vi "Motion-Energize-Drives.vi"(8 "error in (no error)":errorcluster, 11 "Motion-ControlAll in":refnum<class "Motion-ControlAll.lvclass">) -> (0 "error out":errorcluster, 3 "Motion-ControlAll out":refnum<class "Motion-ControlAll.lvclass">)   [LabVIEW 2013, in "Motion-ControlAll.lvclass"]
uses:
  Motion-ControlAll.lvclass
  Motion-ControlAll.lvclass/Motion-ControlAll.ctl
  <vilib>/addons/_LabVIEW Style Book/Utilities/Style Book Utilities.lvlib
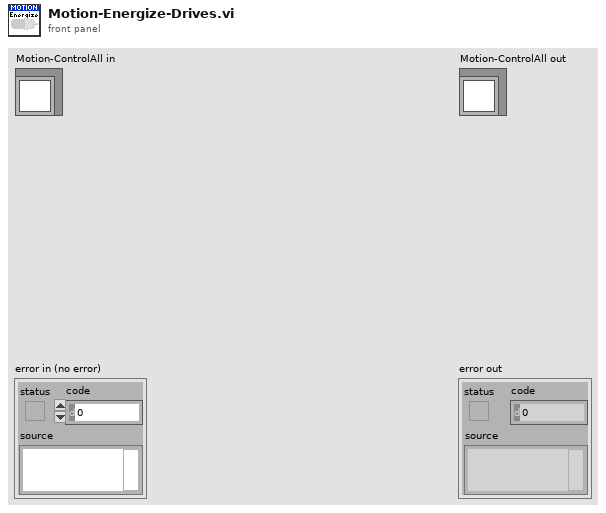
[diagram p1: front panel]
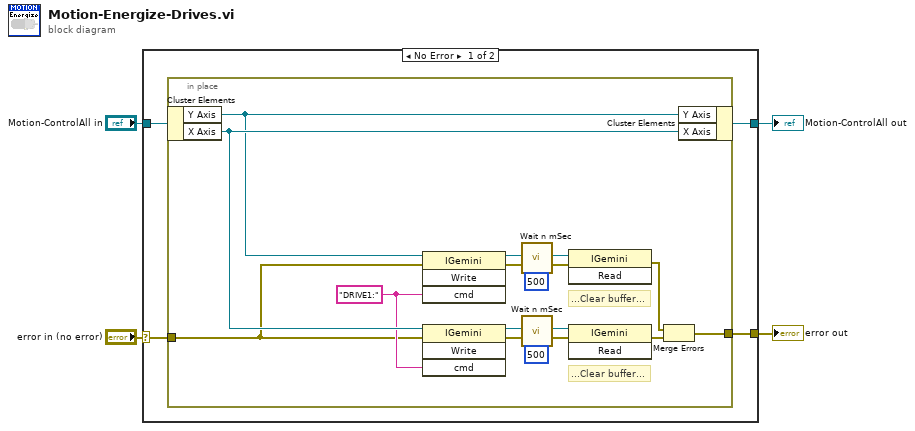
[diagram p0: block diagram]
diagram:
  n1 = case shown="No Error" "error in (no error)" {
    selector: "error in (no error)" -> [w7 w25]
    tunnel: [w6 w25] -> w3
    tunnel: [w5 w24] -> w1
    tunnel: "Motion-ControlAll in" -> [w8 w24]
    frame No Error {
      n2 = in-place {
        in-place-border: w7 -> [w20]
        in-place-border: [w9] -> w6
        w21 = "DRIVE1:"
        # "...Clear buffer..."
        # "...Clear buffer..."
        n3 = in-place-cluster #1(w8) -> ("Y Axis"=w22:refnum<k7>, "X Axis"=w23:refnum<k7>)
        n4 = invoke class="IGemini" method="Write"(reference=w22, error in=w20, "cmd"=w21) -> (reference out=w16:refnum<k7>, error out=w17:errorcluster)  [unwired: 1 in, 2 out]
        n5 = invoke class="IGemini" method="Write"(reference=w23, error in=w20, "cmd"=w21) -> (reference out=w10:refnum<k7>, error out=w12:errorcluster)  [unwired: 1 in, 2 out]
        n6 = call <vilib>:"Wait n mSec.vi"("error in (no error)"=w17, "Milliseconds to Wait (500)"=u32 500) -> ("error out"=w15:errorcluster)  [unwired: 13 in]
        n7 = call <vilib>:"Wait n mSec.vi"("error in (no error)"=w12, "Milliseconds to Wait (500)"=u32 500) -> ("error out"=w11:errorcluster)  [unwired: 13 in]
        n8 = invoke class="IGemini" method="Read"(reference=w16, error in=w15) -> (error out=w18:errorcluster)  [unwired: 1 in, 2 out]
        n9 = invoke class="IGemini" method="Read"(reference=w10, error in=w11) -> (error out=w19:errorcluster)  [unwired: 1 in, 2 out]
        n10 = Merge Errors(w18, w19) -> (w9:errorcluster)
        n11 = in-place-cluster #1("Y Axis"=w22, "X Axis"=w23) -> (w5:refnum<class "Motion-ControlAll.lvclass">)
      }
    }
    frame Error {
    }
  }
  "error out" <- w3
  "Motion-ControlAll out" <- w1
